vi "lvBuildSpec.vi"() -> (0 "error out":errorcluster)   [LabVIEW 2016, in "lvcommonbuild.lvlib"]
uses:
  lvcommonbuild.lvlib
  <vilib>/Wiresmith Technology/LabVIEW CLI/CLI Class/CLI.lvclass
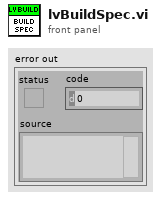
[diagram p1: front panel]
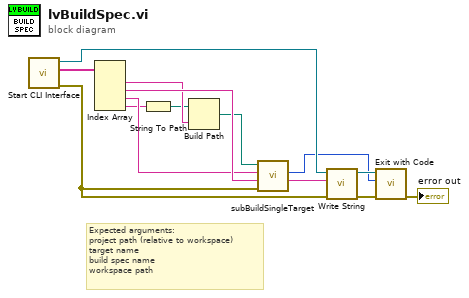
[diagram p0: block diagram]
diagram:
  # "Expected arguments:\nproject path (relative to workspace)\ntarget name\nbuild spec name\nworkspace path"
  n1 = call <vilib>:"Start CLI Interface.vi"() -> ("error out"=w5:errorcluster, "Custom Parameters"=w14:string[], "CLI out"=w12:refnum<class "CLI.lvclass">)  [unwired: 9 in]
  n2 = Index Array(array=w14) -> (element #1=w4:string, element #2=w7:string, element #3=w6:string, element #4=w3:string)  [unwired: 4 in]
  n3 = String To Path(string=w3) -> (path=w2:path)
  n4 = Build Path(base path=w2, name or relative path=w4) -> (appended path=w1:path)
  n5 = call "subBuildSingleTarget.vi"("error in (no error)"=w5, "Target"=w7, "Build Spec"=w6, "Project"=w1) -> ("Output Message"=w13:string, "Exit Code (0)"=w9:i32)  [unwired: 5 in, 1 out]
  n6 = call <vilib>:"Write String.vi"("error in (no error)"=w5, "Text to Write"=w13, "CLI in"=w12) -> ("error out"=w11:errorcluster, "CLI out"=w10:refnum<class "CLI.lvclass">)  [unwired: 7 in]
  n7 = call <vilib>:"Exit with Code.vi"("error in (no error)"=w11, "Exit Code (0)"=w9, "CLI in"=w10) -> ("error out"=→"error out":errorcluster)  [unwired: 8 in]
